vi "Parallel Mode Write.vi"(8 "error in":errorcluster, 10 "Parallel Mode STS":i32, 11 "Cycler in":refnum<class "Cycler.lvclass">) -> (0 "error out":errorcluster, 3 "Cycler out":refnum<class "Cycler.lvclass">)   [LabVIEW 2023, in "Cycler.lvclass"]
uses:
  Cycler.lvclass
  Cycler.lvclass/Cycler.ctl
  Low Level Capabilities/Parallel Mode/Parallel Mode.lvclass
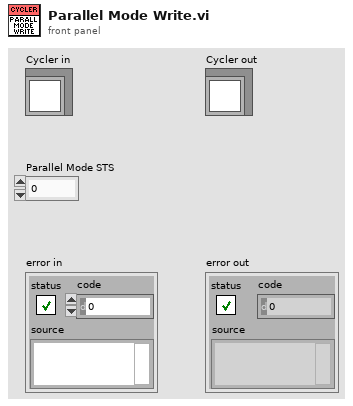
[diagram p1: front panel]
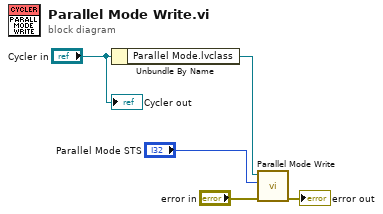
[diagram p0: block diagram]
diagram:
  n1 = Unbundle By Name("Cycler in") -> ("Parallel Mode.lvclass"=w3:refnum<class "Parallel Mode.lvclass">)
  n2 = call-dynamic "Parallel Mode Write.vi"("error in"="error in", "Parallel Mode STS"="Parallel Mode STS", "Parallel Mode in"=w3) -> ("error out"=→"error out":errorcluster)  [unwired: 7 in, 1 out]
  "Cycler out" <- "Cycler in"
